vi "DS11202Z Read Waveform.vi"(10 "通道":enum16{"Channel_1", "Channel_2"}(ring), 11 "TestIndex":i32) -> (0 "错误输出":errorcluster)   [LabVIEW 2015]
panel:
  out "大小":i32
  out "波形图":dbl[](graph)
  out "Data":dbl[](array[numeric])
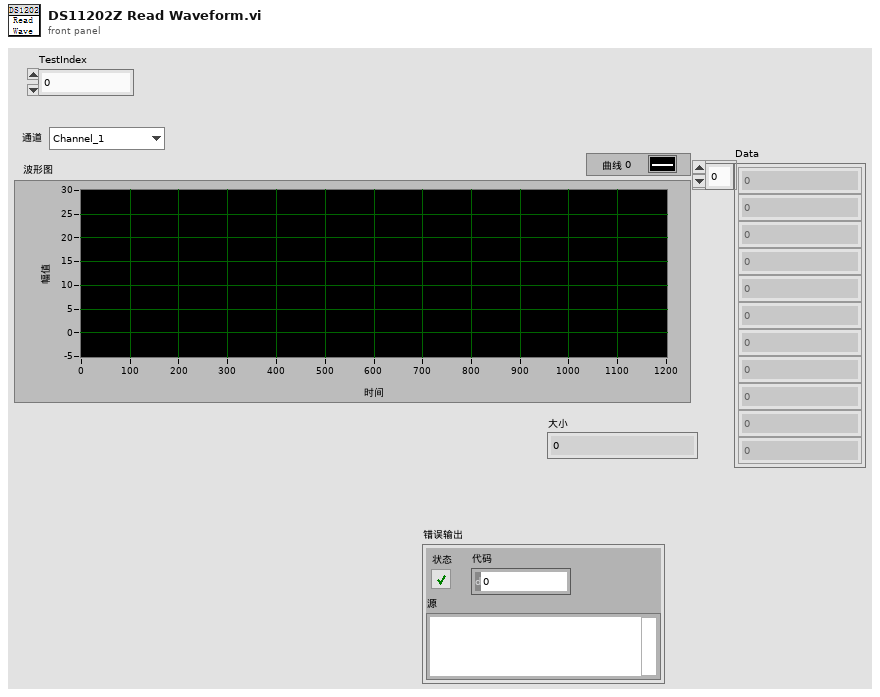
[diagram p1: front panel]
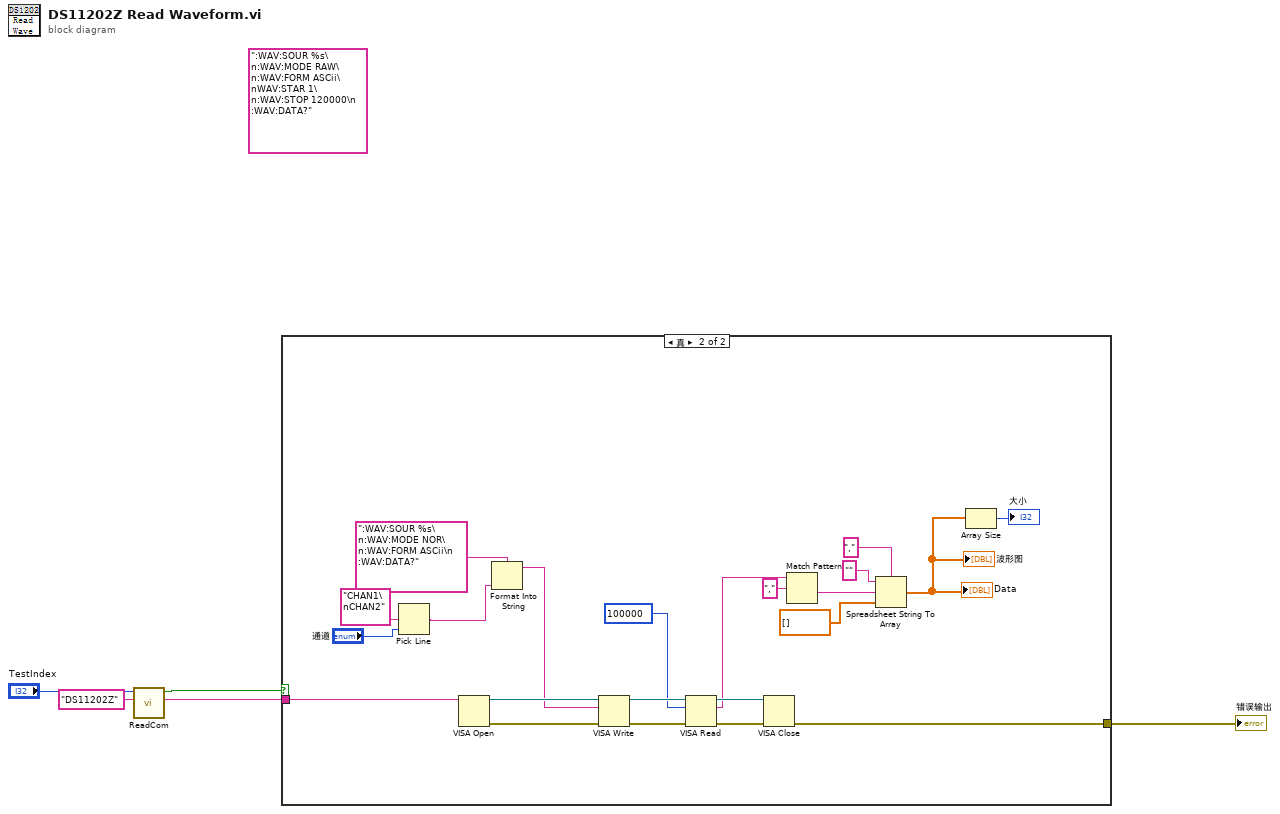
[diagram p0: block diagram]
diagram:
  (unwired) ":WAV:SOUR %s\n:WAV:MODE RAW\n:WAV:FORM ASCii\nWAV:STAR 1\n:WAV:STOP 120000\n :WAV:DATA?" ("字符串")
  n1 = call "ReadCom.vi"("仪器名称"="DS11202Z", "MyIndex"="TestIndex") -> ("COM"=w2:string, "OK?"=w1:bool)  [unwired: 7 in, 1 out]
  n2 = case shown="真" w1 {
    tunnel: [_ w25] -> w5
    tunnel: w2 -> [_ w6]
    frame False {
    }
    frame True {
      n3 = Pick Line(multi-line string="CHAN1\nCHAN2", line index="通道") -> (output string=w7:string)  [unwired: 1 in]
      n4 = VISA Open(VISA resource name=w6) -> (VISA resource name=w27:refnum<visa-resource-name>, error out=w26:errorcluster)  [unwired: 1 in, 3 out]
      n5 = Format Into String(format string=":WAV:SOUR %s\n:WAV:MODE NOR\n:WAV:FORM ASCii\n :WAV:DATA?" ("字符串"), w7) -> (resulting string=w10:string)  [unwired: 2 in, 1 out]
      n6 = VISA Write(VISA resource name=w27, write buffer=w10, error in (no error)=w26) -> (VISA resource name out=w16:refnum<visa-resource-name>, error out=w11:errorcluster)  [unwired: 1 out]
      n7 = VISA Read(VISA resource name=w16, byte count=u32 100000 ("字节总数"), error in (no error)=w11) -> (VISA resource name out=w15:refnum<visa-resource-name>, read buffer=w12:string, error out=w14:errorcluster)  [unwired: 1 out]
      n8 = VISA Close(VISA resource name=w15, error in (no error)=w14) -> (error out=w25:errorcluster)
      n9 = Match Pattern(string=w12, regular expression="," ("正则表达式")) -> (after substring=w19:string)  [unwired: 1 in, 3 out]
      n10 = Spreadsheet String To Array(delimiter (Tab)="," ("分隔符(Tab)"), format string="" ("格式字符串"), spreadsheet string=w19, array type (2D Dbl)=dbl[] []) -> (array=w18:dbl[])
      "Data" <- w18
      "波形图" <- w18
      n11 = Array Size(array=w18) -> (size(s)=→"大小":i32)
    }
  }
  "错误输出" <- w5
